vi "P116ComandoSecuencia.vi"(9 "RateSP":T1, 10 "NuevoSP":T1) -> (1 "RateSP(C/min) 2":T1, 2 "NuevoSP(C) 2":T1, 3 "Cancel 2":bool)   [LabVIEW 2013]
uses:
  3xP116.ctl
panel:
  in  "Cancel":bool
  in  "Write":bool
  # "Controladores P116"
  # "C"
  # "ARRIBA"
  # "C/min"
  # "C"
  # "ABAJO"
  # "C/min"
  # "C"
  # "CINTAS"
  # "C/min"
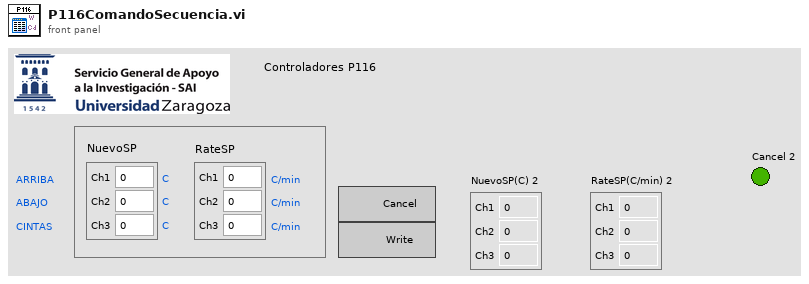
[diagram p1: front panel]
types:
  T1 = typedef "3xP116.ctl" = cluster{"Ch1":dbl, "Ch2":dbl, "Ch3":dbl}
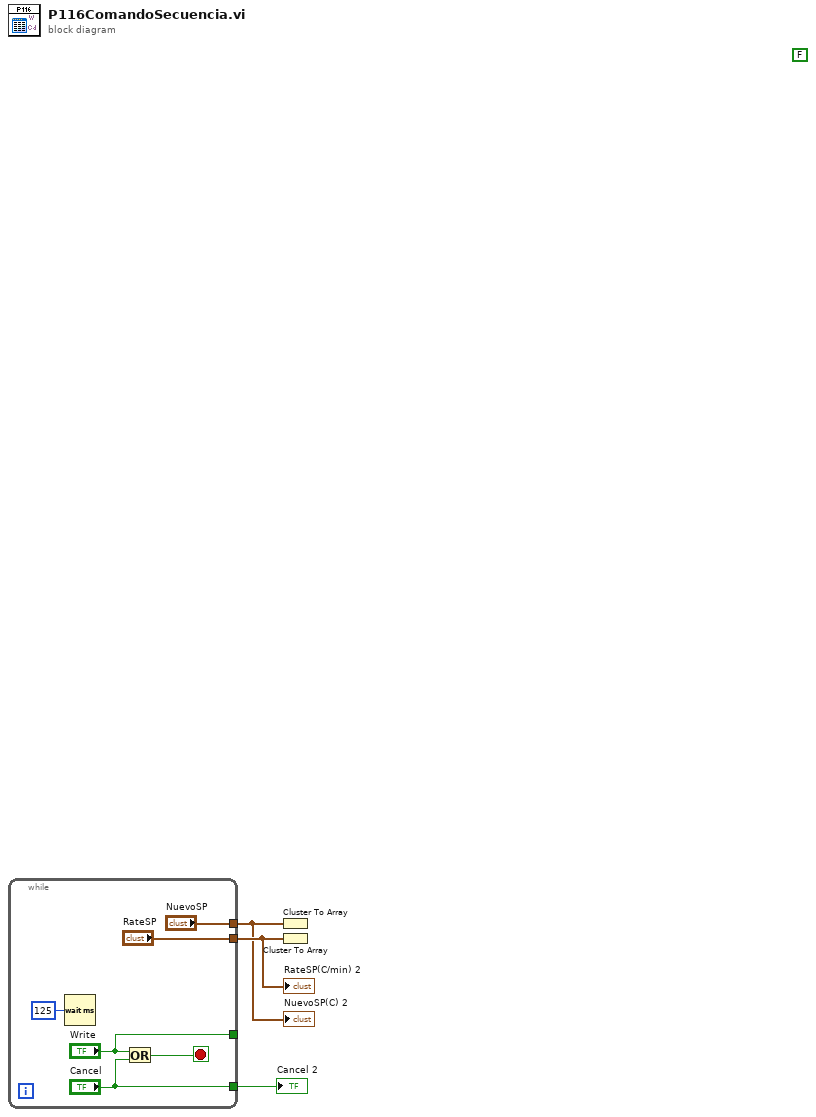
[diagram p0: block diagram]
diagram:
  (unwired) FALSE
  n1 = while {
    tunnel: ["Cancel"] -> w1
    tunnel: ["NuevoSP"] -> w2
    tunnel: ["RateSP"] -> w3
    tunnel: ["Write"] -> _
    stop <- w4 stop-if-true
    n2 = Wait (ms)(milliseconds to wait=u32 125) -> ()  [unwired: 1 out]
    n3 = Or(x="Write", y="Cancel") -> (x .or. y?=w4:bool)
  }
  "NuevoSP(C) 2" <- w2
  "RateSP(C/min) 2" <- w3
  "Cancel 2" <- w1
  n4 = Cluster To Array(cluster=w2) -> ()  [unwired: 1 out]
  n5 = Cluster To Array(cluster=w3) -> ()  [unwired: 1 out]
